vi "ex8-4.vi"   [LabVIEW 2009]
uses:
  <vilib>/NXT/Dual Mode Library/Display/NXT_Rect.ctl
  <vilib>/NXT/Dual Mode Library/Waits/Wait_Num.vi
  <vilib>/NXT/Dual Mode Library/Display/drawPoint.vi
  <vilib>/NXT/Dual Mode Library/Display/drawRect.vi
  <vilib>/NXT/Dual Mode Library/Display/drawLine.vi
  <vilib>/NXT/Dual Mode Library/Display/drawCircle.vi
types:
  T1 = cluster{"Origin X":i16, "Origin Y":i16, "Radius":u8}
  T2 = cluster{"Start X":i16, "Start  Y":i16, "End X":i16, "End Y":i16}
  T3 = typedef "NXT_Rect.ctl" = cluster{"Left":i16, "Bottom":i16, "Width":i16, "Height":i16}
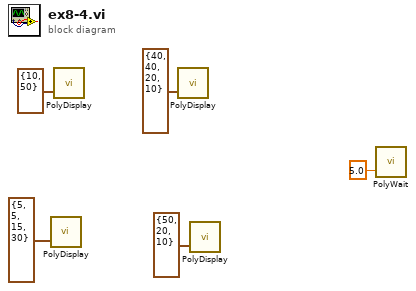
[diagram p0: block diagram]
diagram:
  n1 = call-poly <vilib>:"PolyDisplay.vi"("Line Parameters"=T2 {"Start X"=5, "Start  Y"=5, "End X"=15, "End Y"=30}) -> ()  [unwired: 3 in, 1 out]
  n2 = call-poly <vilib>:"PolyDisplay.vi"("Coordinates"=cluster{"X":i16, "Y":i16} {"X"=10, "Y"=50}) -> ()  [unwired: 3 in, 1 out]
  n3 = call-poly <vilib>:"PolyDisplay.vi"("Rect Parameters"=T3 {"Left"=40, "Bottom"=40, "Width"=20, "Height"=10}) -> ()  [unwired: 3 in, 1 out]
  n4 = call-poly <vilib>:"PolyDisplay.vi"("Circle Parameters"=T1 {"Origin X"=50, "Origin Y"=20, "Radius"=10}) -> ()  [unwired: 3 in, 1 out]
  n5 = call-poly <vilib>:"PolyWait.vi"("Time (1 sec)"=sgl 5.0) -> ()  [unwired: 3 in, 1 out]
